vi "pruebas.vi"   [LabVIEW 2013, in "Proyecto 2 Touch.lvrbt"]
uses:
  Proyecto 2 Touch.lvrbt
  <vilib>/NXT/Block Support/NXT_OutputPort.ctl
  <vilib>/NXT/Dual Mode Library/Waits/Wait_Rotation.vi
  <vilib>/NXT/Dual Mode Library/Waits/Wait_Num.vi
  <vilib>/NXT/NXTIO Xnodes/NXTIONodeSubVIs/LEGOResetMotors.vi
  <vilib>/NXT/NXTIO Xnodes/NXTIONodeSubVIs/NXTMoveMotors.vi
  <vilib>/NXT/NXTIO Xnodes/NXTIONodeSubVIs/LEGOStopAllMotors.vi
  <vilib>/NXT/Subs/LVHSConnector.ctl
  <vilib>/NXT/NXTIO Xnodes/AddressXNode/NXTIOAddress.xnode
  <vilib>/NXT/NXTIO Xnodes/NXTIOXNode/NXTIO.xnode
  <vilib>/NXT/LegoClasses/BrickReference/BrickReference.lvclass
types:
  T1 = typedef "NXT_OutputPort.ctl" = u8
  T2 = typedef "LVHSConnector.ctl" = refnum<class "BrickReference.lvclass">
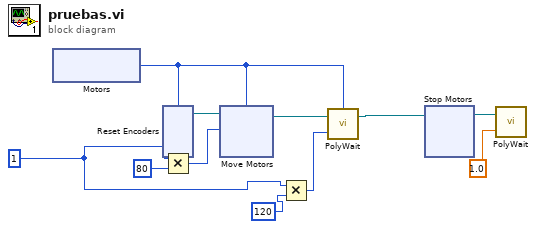
[diagram p0: block diagram]
diagram:
  w4 = 1 ("x")
  n1 = xnode "Motors"() -> ("Motor"=w3:T1)
  n2 = xnode "Reset Encoders"("Motors"=w3) -> ("NXT/EV3"=w10:T2)  [unwired: 1 in]
  n3 = Multiply(x=w4, y=80) -> (x*y=w6:i32)
  n4 = xnode "Move Motors"("Power/Speed 1"=w6, "Motors"=w3, "NXT/EV3"=w10) -> ("NXT/EV3"=w7:T2)
  n5 = Multiply(x=w4, y=120) -> (x*y=w5:i32)
  n6 = call-poly <vilib>:"PolyWait.vi"("Position Change (180)"=w5, "NXT/EV3"=w7, "Port (Port A)"=w3) -> ("NXT/EV3"=w2:T2)  [unwired: 1 in]
  n7 = xnode "Stop Motors"("NXT/EV3"=w2) -> ("NXT/EV3"=w9:T2)  [unwired: 1 in]
  n8 = call-poly <vilib>:"PolyWait.vi"("Time (1 sec)"=sgl 1.0, "NXT/EV3"=w9) -> ()  [unwired: 2 in, 1 out]
